vi "Write LabVIEWHTTPClient_NET.vi"(8 "error in (no error)":errorcluster, 10 "LabVIEWHTTPClient_NET.lvlib:LabVIEWHTTPClient_NET":refnum<class "LabVIEWHTTPClient_NET.lvclass">, 11 "REST Client_NET in":refnum<class "REST Client_NET.lvclass">) -> (0 "error out":errorcluster, 3 "REST Client_NET out":refnum<class "REST Client_NET.lvclass">)   [LabVIEW 2018, in "REST Client_NET.lvlib" / "REST Client_NET.lvclass"]
uses:
  REST Client_NET.lvclass
  LabVIEWHTTPClient_NET/LabVIEWHTTPClient_NET.lvclass
  REST Client_NET.lvclass/REST Client_NET.ctl
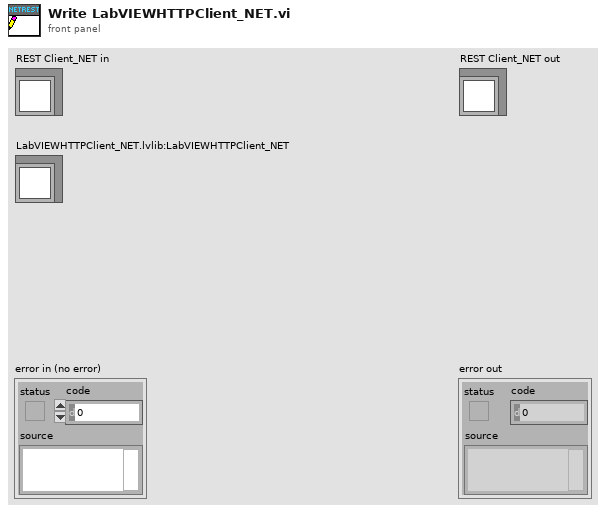
[diagram p1: front panel]
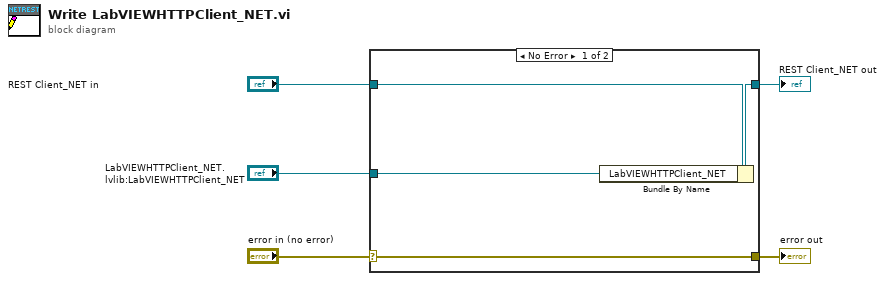
[diagram p0: block diagram]
diagram:
  n1 = case shown="No Error" "error in (no error)" {
    selector: "error in (no error)" -> [w9 w10]
    tunnel: [w9 w10] -> w4
    tunnel: [w7 w11] -> w2
    tunnel: "REST Client_NET in" -> [w8 w11]
    tunnel: "LabVIEWHTTPClient_NET.lvlib:LabVIEWHTTPClient_NET" -> [w6 _]
    frame No Error {
      n2 = Bundle By Name(cluster=w8, "LabVIEWHTTPClient_NET"=w6) -> (w7:refnum<class "REST Client_NET.lvclass">)
    }
    frame Error {
    }
  }
  "error out" <- w4
  "REST Client_NET out" <- w2
